vi "parseReportServerIDFrame.vi"(8 "error in (no error)":errorcluster, 10 "ModbusBuffer in":refnum<class "ModbusBuffer.lvclass">, 11 "ILC in":refnum<class "ILC.lvclass">) -> (0 "error out":errorcluster, 2 "ModbusBuffer out":refnum<class "ModbusBuffer.lvclass">, 3 "ILC out":refnum<class "ILC.lvclass">)   [LabVIEW 2016, in "RTILC.lvlib" / "ILC.lvclass"]
uses:
  ILC.lvclass
  Common_RT_Modbus/ModbusBuffer/ModbusBuffer.lvclass
  Common_RT_Modbus/ModbusBuffer/ModbusBuffer.lvclass/ModbusBuffer.ctl
  Common_RT_Modbus/DataTypes/ExceptionCodes.ctl
  ILC.lvclass/ILC.ctl
  Common_RT_Modbus/ModbusBuffer/readTimestampByte.vi
  Common_RT_Modbus/ModbusBuffer/readInstructionByte.vi
  Common_RT_Modbus/RTModbus.lvlib
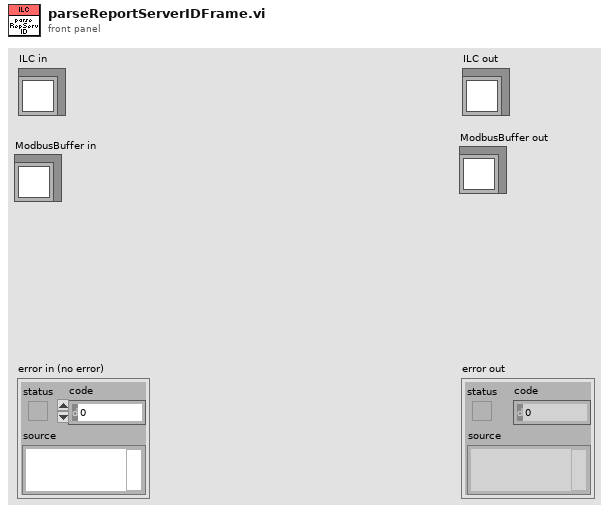
[diagram p1: front panel]
types:
  T1 = typedef "RTModbus.lvlib/ExceptionCodes.ctl" = u16
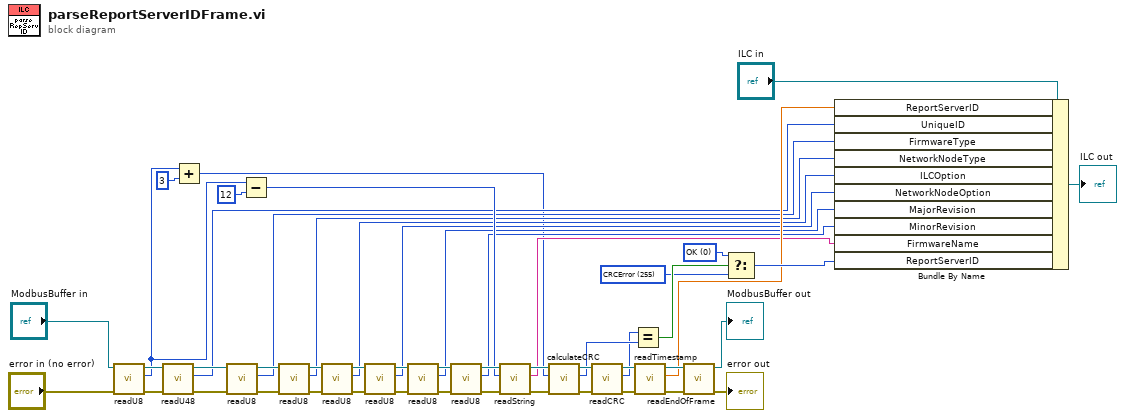
[diagram p0: block diagram]
diagram:
  w46 = T1 255 items=["OK"=0, "IllegalFunction"=1, "IllegalDataAddress"=2, "IllegalDataValue"=3, "SlaveDeviceFailure"=4, "Acknowledge"=5, "SlaveDeviceBusy"=6, "NegativeAcknowledge"=7, "MemoryParityError"=8, "GatewayPathUnavailable"=9, "GatewayTargetDeviceFailedToRespond"=10, "WaitingForResponse"=254, "CRCError"=255] ("f")
  w47 = T1 0 items=["OK"=0, "IllegalFunction"=1, "IllegalDataAddress"=2, "IllegalDataValue"=3, "SlaveDeviceFailure"=4, "Acknowledge"=5, "SlaveDeviceBusy"=6, "NegativeAcknowledge"=7, "MemoryParityError"=8, "GatewayPathUnavailable"=9, "GatewayTargetDeviceFailedToRespond"=10, "WaitingForResponse"=254, "CRCError"=255] ("Responses.ADCOffsetSensitivity")
  n1 = call "readU8.vi"("error in (no error)"="error in (no error)", "ModbusBuffer in"="ModbusBuffer in") -> ("error out"=w19:errorcluster, "Output"=w3:u8, "ModbusBuffer out"=w36:refnum<class "ModbusBuffer.lvclass">)  [unwired: 7 in]
  n2 = call "readU48.vi"("error in (no error)"=w19, "ModbusBuffer in"=w36) -> ("error out"=w20:errorcluster, "Output"=w4:u64, "ModbusBuffer out"=w35:refnum<class "ModbusBuffer.lvclass">)  [unwired: 7 in]
  n3 = Add(x=w3, y=u8 3) -> (x+y=w1:u8)
  n4 = call "readU8.vi"("error in (no error)"=w20, "ModbusBuffer in"=w35) -> ("error out"=w21:errorcluster, "Output"=w5:u8, "ModbusBuffer out"=w34:refnum<class "ModbusBuffer.lvclass">)  [unwired: 7 in]
  n5 = Subtract(x=w3, y=u8 12) -> (x-y=w11:u8)
  n6 = call "readU8.vi"("error in (no error)"=w21, "ModbusBuffer in"=w34) -> ("error out"=w22:errorcluster, "Output"=w6:u8, "ModbusBuffer out"=w33:refnum<class "ModbusBuffer.lvclass">)  [unwired: 7 in]
  n7 = call "readU8.vi"("error in (no error)"=w22, "ModbusBuffer in"=w33) -> ("error out"=w23:errorcluster, "Output"=w7:u8, "ModbusBuffer out"=w32:refnum<class "ModbusBuffer.lvclass">)  [unwired: 7 in]
  n8 = call "readU8.vi"("error in (no error)"=w23, "ModbusBuffer in"=w32) -> ("error out"=w24:errorcluster, "Output"=w8:u8, "ModbusBuffer out"=w31:refnum<class "ModbusBuffer.lvclass">)  [unwired: 7 in]
  n9 = call "readU8.vi"("error in (no error)"=w24, "ModbusBuffer in"=w31) -> ("error out"=w25:errorcluster, "Output"=w9:u8, "ModbusBuffer out"=w30:refnum<class "ModbusBuffer.lvclass">)  [unwired: 7 in]
  n10 = call "readU8.vi"("error in (no error)"=w25, "ModbusBuffer in"=w30) -> ("error out"=w26:errorcluster, "Output"=w10:u8, "ModbusBuffer out"=w29:refnum<class "ModbusBuffer.lvclass">)  [unwired: 7 in]
  n11 = call "readString.vi"("error in (no error)"=w26, "Length"=w11, "ModbusBuffer in"=w29) -> ("error out"=w27:errorcluster, "Output"=w13:string, "ModbusBuffer out"=w28:refnum<class "ModbusBuffer.lvclass">)  [unwired: 6 in]
  n12 = call "calculateCRC.vi"("error in (no error)"=w27, "Length"=w1, "ModbusBuffer in"=w28) -> ("error out"=w40:errorcluster, "CRC"=w39:u16, "ModbusBuffer out"=w45:refnum<class "ModbusBuffer.lvclass">)  [unwired: 6 in]
  n13 = call "readCRC.vi"("error in (no error)"=w40, "ModbusBuffer in"=w45) -> ("error out"=w41:errorcluster, "Output"=w38:u16, "ModbusBuffer out"=w44:refnum<class "ModbusBuffer.lvclass">)  [unwired: 7 in]
  n14 = Equal?(x=w38, y=w39) -> (x = y?=w48:bool)
  n15 = call "readTimestamp.vi"("error in (no error)"=w41, "ModbusBuffer in"=w44) -> ("error out"=w42:errorcluster, "Output"=w14:dbl, "ModbusBuffer out"=w43:refnum<class "ModbusBuffer.lvclass">)  [unwired: 7 in]
  n16 = call "readEndOfFrame.vi"("error in (no error)"=w42, "ModbusBuffer in"=w43) -> ("error out"=→"error out":errorcluster, "ModbusBuffer out"=→"ModbusBuffer out":refnum<class "ModbusBuffer.lvclass">)  [unwired: 8 in]
  n17 = Select(t=w47, s=w48, f=w46) -> (s? t:f=w15:T1)
  n18 = Bundle By Name(cluster="ILC in", "ReportServerID"=w14, "UniqueID"=w4, "FirmwareType"=w5, "NetworkNodeType"=w6, "ILCOption"=w7, "NetworkNodeOption"=w8, "MajorRevision"=w9, "MinorRevision"=w10, "FirmwareName"=w13, "ReportServerID"=w15) -> (→"ILC out":refnum<class "ILC.lvclass">)
